vi "Read guideStateTypes.vi"(8 "error in (no error)":errorcluster, 11 "Guide in":refnum<class "Guide.lvclass">) -> (0 "error out":errorcluster, 2 "guideStateTypes":T1, 3 "Guide out":refnum<class "Guide.lvclass">)   [LabVIEW 2022 SP3, in "TCSDataDefinitions.lvlib" / "TCSCommand.lvlib" / "GuiderCommands.lvlib" / "Guide.lvclass"]
uses:
  Guide.lvclass
  Enumerations/GuideStateTypes.ctl
  Guide.lvclass/Guide.ctl
  TCSCommand.lvlib
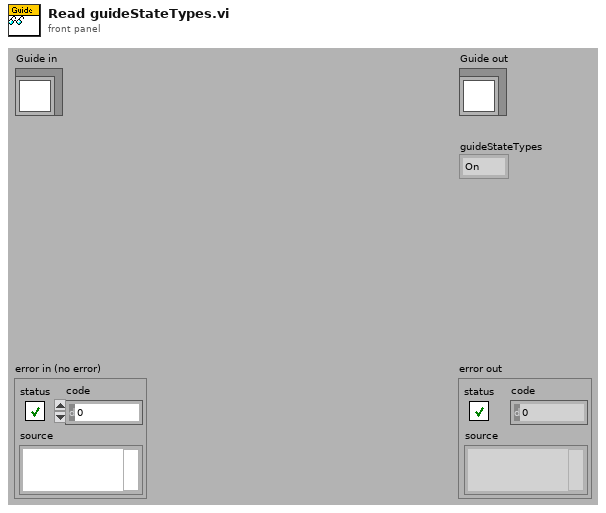
[diagram p1: front panel]
types:
  T1 = typedef "TCSDataDefinitions.lvlib/TCSCommand.lvlib/GuideStateTypes.ctl" = enum16{"On", "Off"}
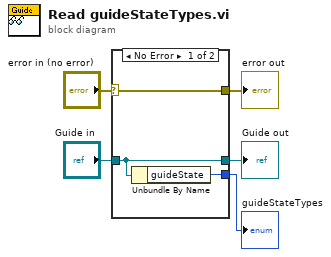
[diagram p0: block diagram]
diagram:
  n1 = case shown="No Error" "error in (no error)" {
    selector: "error in (no error)" -> [w8 w9]
    tunnel: [w8 w9] -> w4
    tunnel: [w7 w10] -> w2
    tunnel: "Guide in" -> [w7 w10]
    tunnel: [w6 _] -> w1
    frame No Error {
      n2 = Unbundle By Name(w7) -> ("guideState"=w6:T1)
    }
    frame Error {
    }
  }
  "error out" <- w4
  "Guide out" <- w2
  "guideStateTypes" <- w1
